vi "parmsQSB.vi"(1 "dimensions":i64[](array[numeric])=[1399090569999999999, -1], 2 "values":T2(array[cluster]), 3 "label":string="parms") -> (0 "JSON string":string="{\"label\":\"parms\",\"values\":[{\"Nchannel\":96,\"ADCbits\":16,\"BridgeVoltage (V)\":5,\"ExptSampleFrequency (Hz)\":1250,\"CalSampleFrequency (Hz)\":1250,\"CalStep1 (V)\":\"2.5\",\"CalStep2 (V)\":\"3.7\",\"detector\":\"Au_Kapton\"}],\"dimensions\":[1399090569999999999,-1]}")   [LabVIEW 2014]
panel:
  out "json string cluster":T1
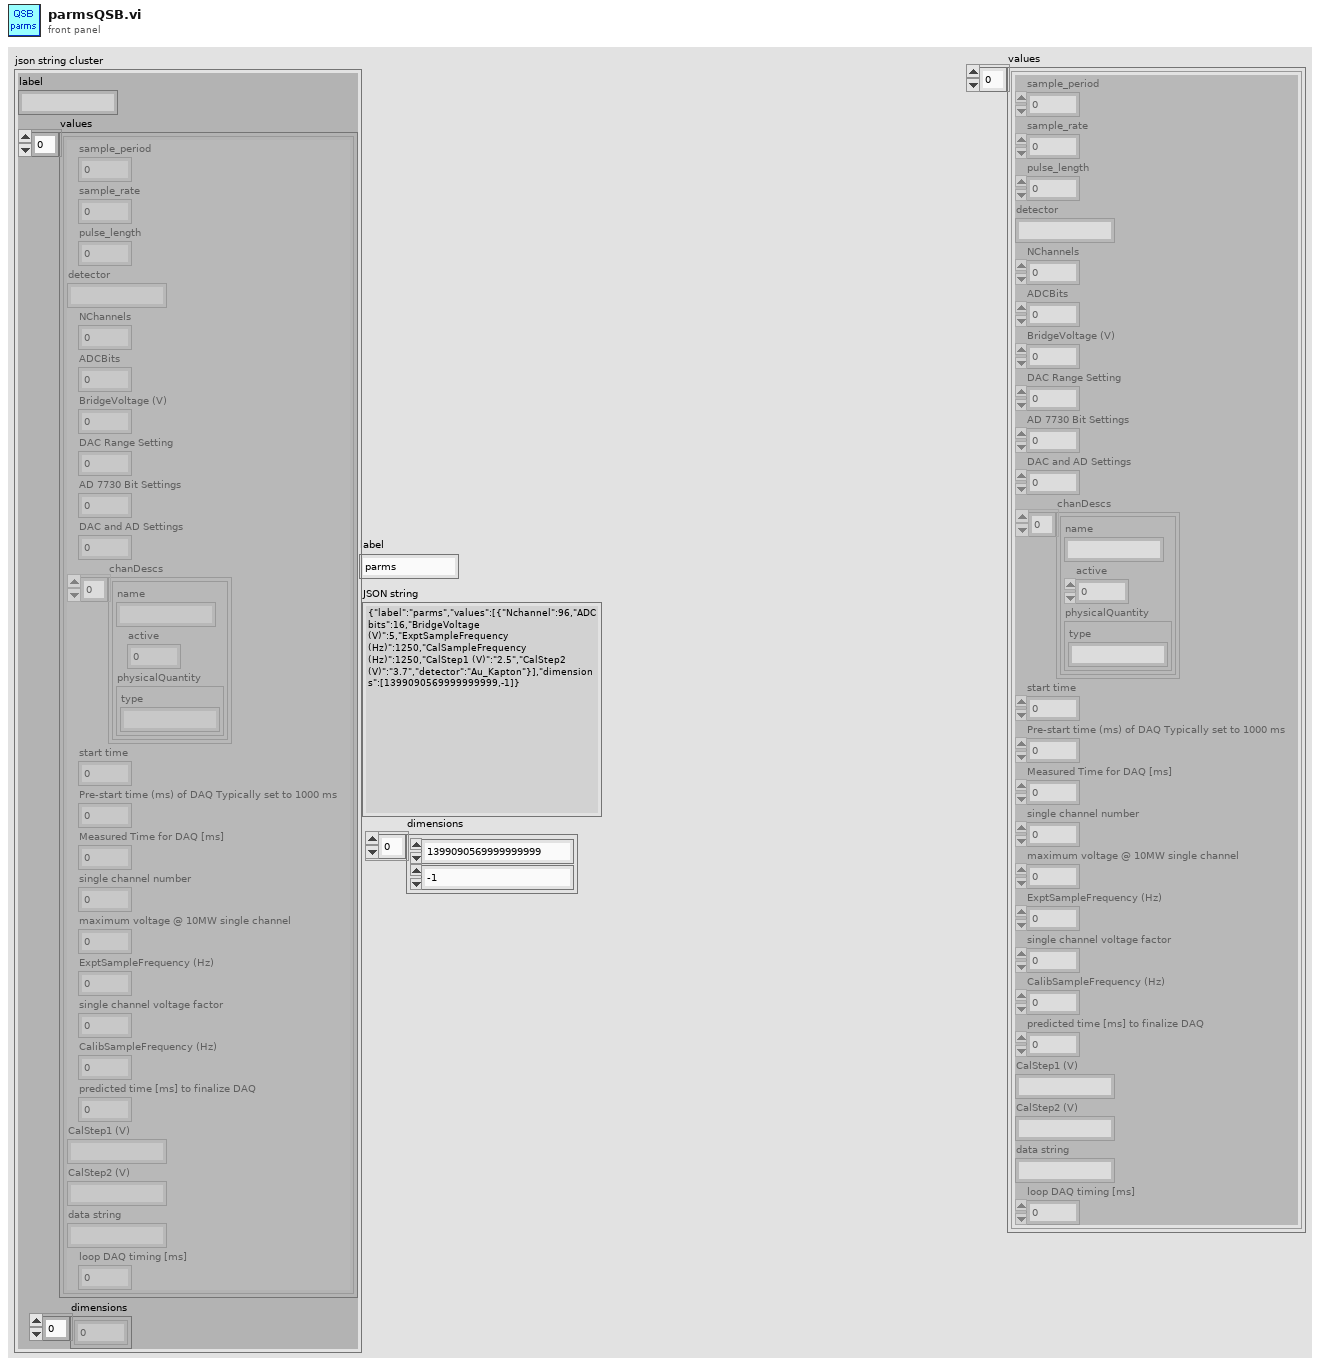
[diagram p1: front panel]
types:
  T1 = cluster{"label":string, "values":cluster{"sample_period":dbl, "sample_rate":dbl, "pulse_length":dbl, "detector":string, "NChannels":i16, "ADCBits":i16, "BridgeVoltage (V)":sgl, "DAC Range Setting":u8, "AD 7730 Bit Settings":i32, "DAC and AD Settings":i32, "chanDescs":cluster{"name":string, "active":i32, "physicalQuantity":cluster{"type":string}}[], "start time":i64, "Pre-start time (ms) of DAQ Typically set to 1000 ms":i32, "Measured Time for DAQ [ms] ":u32, "single channel number":i64, "maximum voltage @ 10MW single channel":dbl, "ExptSampleFrequency (Hz)":sgl, "single channel voltage factor":dbl, "CalibSampleFrequency (Hz)":sgl, "predicted time [ms] to finalize DAQ":dbl, "CalStep1 (V)":string, "CalStep2 (V)":string, "data string":string, "loop DAQ timing [ms]":dbl}[], "dimensions":i64[]}
  T2 = cluster{"sample_period":dbl, "sample_rate":dbl, "pulse_length":dbl, "detector":string, "NChannels":i16, "ADCBits":i16, "BridgeVoltage (V)":sgl, "DAC Range Setting":u8, "AD 7730 Bit Settings":i32, "DAC and AD Settings":i32, "chanDescs":cluster{"name":string, "active":i32, "physicalQuantity":cluster{"type":string}}[], "start time":i64, "Pre-start time (ms) of DAQ Typically set to 1000 ms":i32, "Measured Time for DAQ [ms] ":u32, "single channel number":i64, "maximum voltage @ 10MW single channel":dbl, "ExptSampleFrequency (Hz)":sgl, "single channel voltage factor":dbl, "CalibSampleFrequency (Hz)":sgl, "predicted time [ms] to finalize DAQ":dbl, "CalStep1 (V)":string, "CalStep2 (V)":string, "data string":string, "loop DAQ timing [ms]":dbl}[]
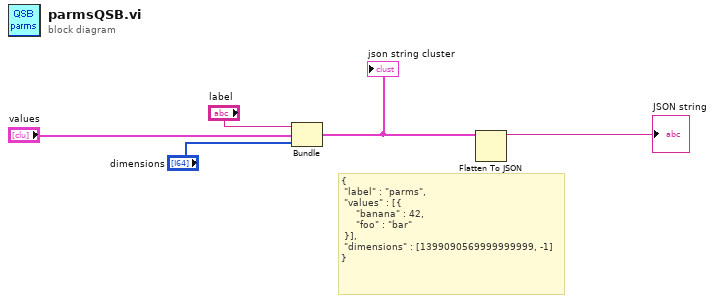
[diagram p0: block diagram]
diagram:
  # "{\n \"label\" : \"parms\",\n \"values\" : [{\n     \"banana\" : 42,\n     \"foo\" : \"bar\"\n }],\n \"dimensions\" : [1399090569999999999, -1]\n}"
  n1 = Bundle("label"="label", "values"="values", "dimensions"="dimensions") -> (w2:T1)  [unwired: 1 in]
  "json string cluster" <- w2
  n2 = Flatten To JSON(anything=w2) -> (JSON string=→"JSON string":string)  [unwired: 2 in, 1 out]
